vi "Read PortSettings.vi"(8 "error in (no error)":errorcluster, 11 "RS232 in":refnum<class "RS-xxx.lvclass">) -> (0 "error out":errorcluster, 2 "PortSettings":T1={"Port"="COM1", "Baud Rate"=9600, "Data Bits"=8, "Parity"=enum."None", "Stop Bits"=10, "Flow Control"=0, "XON"=enum."DC1", "XOFF"=enum."DC3", "End Read on Termination Character"=TRUE, "End Write on Termination Character"=TRUE, "Termination Character"=10, "4wireMode"=TRUE, "AssertDTR"=TRUE, "WireMode"=-1} {"WireMode" items=["Unknown"=-1, "RS485/Wire4"=0, "RS485/Wire2-EchoDTR"=1, "RS485/Wire2-CtrlDTR"=2, "RS485/Wire2-Auto"=3, "RS232/DTE"=128, "RS232/DCE"=129, "RS232/Auto"=130]; "Termination Character" format="%.0x"; "Flow Control" items=["None"=0, "XON/XOFF"=1, "RTS/CTS"=2, "DTR/DSR"=4]; "Stop Bits" items=["1.0"=10, "1.5"=15, "2.0"=20]; "Data Bits" min=5 max=8 step=1; "Baud Rate" items=["75"=75, "110"=110, "134"=134, "150"=150, "300"=300, "600"=600, "1200"=1200, "1800"=1800, "2400"=2400, "4800"=4800, "7200"=7200, "9600"=9600, "14400"=14400, "19200"=19200, "28800"=28800, "38400"=38400, "56000"=56000, "57600"=57600, "115200"=115200, "128000"=128000, "230400"=230400]}, 3 "RS232 out":refnum<class "RS-xxx.lvclass">)   [LabVIEW 2023, in "Protocols.lvlib" / "RS-xxx.lvclass"]
uses:
  RS-xxx.lvclass
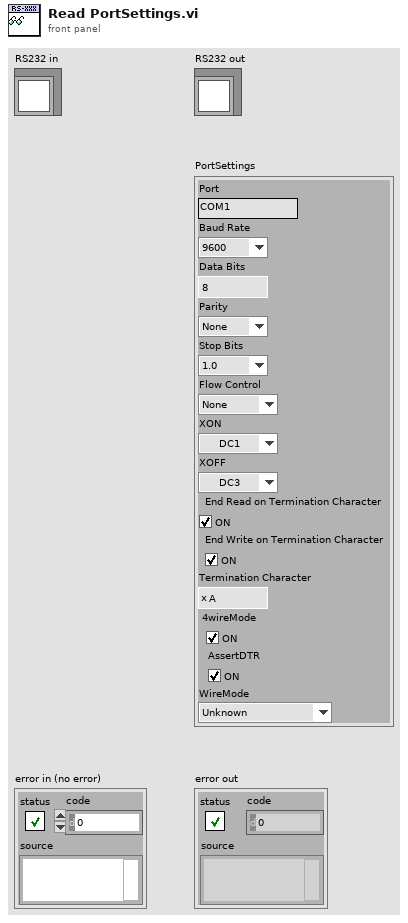
[diagram p1: front panel]
types:
  T1 = cluster{"Port":string, "Baud Rate":u32, "Data Bits":u16, "Parity":enum16{"None", "Odd", "Even", "Mark", "Space"}, "Stop Bits":u16, "Flow Control":u16, "XON":enum16{"NUL", "SOH", "STX", "ETX", "EOT", "ENQ", "ACK", "BEL", "BS", "HT", "LF", "VT", "FF", "CR", "SO", "SI", "DLE", "DC1", "DC2", "DC3", "DC4", "NAK", "SYN", "ETB", "CAN", "EM", "SUB", "ESC", "FS", "GS", "RS", "US", "SP", "!", "\"", "#", "$", "%", "&", "'", "(", ")", "*", "+", ",", "- (-)", ".", "/", "0", "1", "2", "3", "4", "5", "6", "7", "8", "9", ":", ";", "<", "=", ">", "?", "@", "A", "B", "C", "D", "E", "F", "G", "H", "I", "J", "K", "L", "M", "N", "O", "P", "Q", "R", "S", "T", "U", "V", "W", "X", "Y", "Z", "[", "\\", "]", "^", "_", "`", "a", "b", "c", "d", "e", "f", "g", "h", "i", "j", "k", "l", "m", "n", "o", "p", "q", "r", "s", "t", "u", "v", "w", "x", "y", "z", "{", "|", "}", "~"}, "XOFF":enum16{"NUL", "SOH", "STX", "ETX", "EOT", "ENQ", "ACK", "BEL", "BS", "HT", "LF", "VT", "FF", "CR", "SO", "SI", "DLE", "DC1", "DC2", "DC3", "DC4", "NAK", "SYN", "ETB", "CAN", "EM", "SUB", "ESC", "FS", "GS", "RS", "US", "SP", "!", "\"", "#", "$", "%", "&", "'", "(", ")", "*", "+", ",", "- (-)", ".", "/", "0", "1", "2", "3", "4", "5", "6", "7", "8", "9", ":", ";", "<", "=", ">", "?", "@", "A", "B", "C", "D", "E", "F", "G", "H", "I", "J", "K", "L", "M", "N", "O", "P", "Q", "R", "S", "T", "U", "V", "W", "X", "Y", "Z", "[", "\\", "]", "^", "_", "`", "a", "b", "c", "d", "e", "f", "g", "h", "i", "j", "k", "l", "m", "n", "o", "p", "q", "r", "s", "t", "u", "v", "w", "x", "y", "z", "{", "|", "}", "~"}, "End Read on Termination Character":bool, "End Write on Termination Character":bool, "Termination Character":u8, "4wireMode":bool, "AssertDTR":bool, "WireMode":i16}
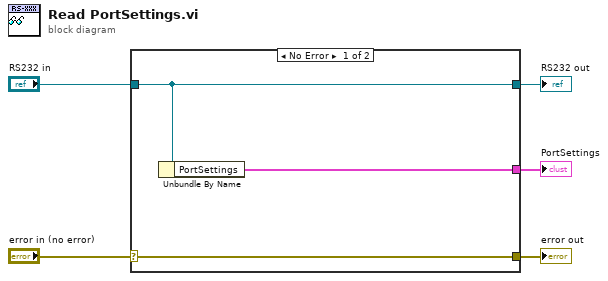
[diagram p0: block diagram]
diagram:
  n1 = case shown="No Error" "error in (no error)" {
    selector: "error in (no error)" -> [w8 w9]
    tunnel: [w8 w9] -> w4
    tunnel: [w7 w10] -> w2
    tunnel: "RS232 in" -> [w7 w10]
    tunnel: [w6 _] -> w1
    frame No Error {
      n2 = Unbundle By Name(w7) -> ("PortSettings"=w6:T1)
    }
    frame Error {
    }
  }
  "error out" <- w4
  "RS232 out" <- w2
  "PortSettings" <- w1
